vi "8-Axis (Producer Consumer - PC).vi"() -> ()   [LabVIEW 2013]
uses:
  Typedef/Typedef_Motor_Message.ctl
  EMC API/EMC_Typedef_Motor_Parameters.ctl
  Functional_Global/Typedef_Message_Queue_Action.ctl
  Globals/Global Stop.vi
  <vilib>/Motion/Express/_s/nimc.ex.clearFaults.clearFaults.axis.vi
  <vilib>/Motion/Express/_s/nimc.ex.power.power.axis.vi
  <vilib>/Motion/Express/_s/nimc.ex.resetPosition.resetPosition.axis.vi
  <vilib>/Motion/Express/_s/nimc.ex.read.readTrajectoryData.axis.vi
  <vilib>/Motion/BlockNode/FB.NIMotion.xnode
  Functional_Global/Typedef_FPGA_Interface_Action.ctl
panel:
  out "Command":T1={"Axis"="", "Motion Parameters"={"position"=1000.0, "velocity"=1000.0, "acceleration"=10000.0, "deceleration"=10000.0, "accel. jerk"=10000.0, "decel. jerk"=10000.0}}
  out "Message":string
  out "# elements in queue":i32
  out "error out":errorcluster
  out "Axis Positions":T3(graph)
  out "Axis Velocities":T3(graph)
  out "Array":dbl[](array[knob]) scale=0.0..1000.0
  in  "stop":bool
  # "This example demonstrates how to set up an multi-axis SW architecture using SoftMotion.  You can have state machines that \"produce\" the motion commands, and the consumer will then digest them one at a time.\n\nIn this example, 3 producer loops generate random motion commands at random times (within 1000ms each iteration.) This VI is also meant as a stress test to see if the SM engine is robust enough for complex sequences of motion commands."
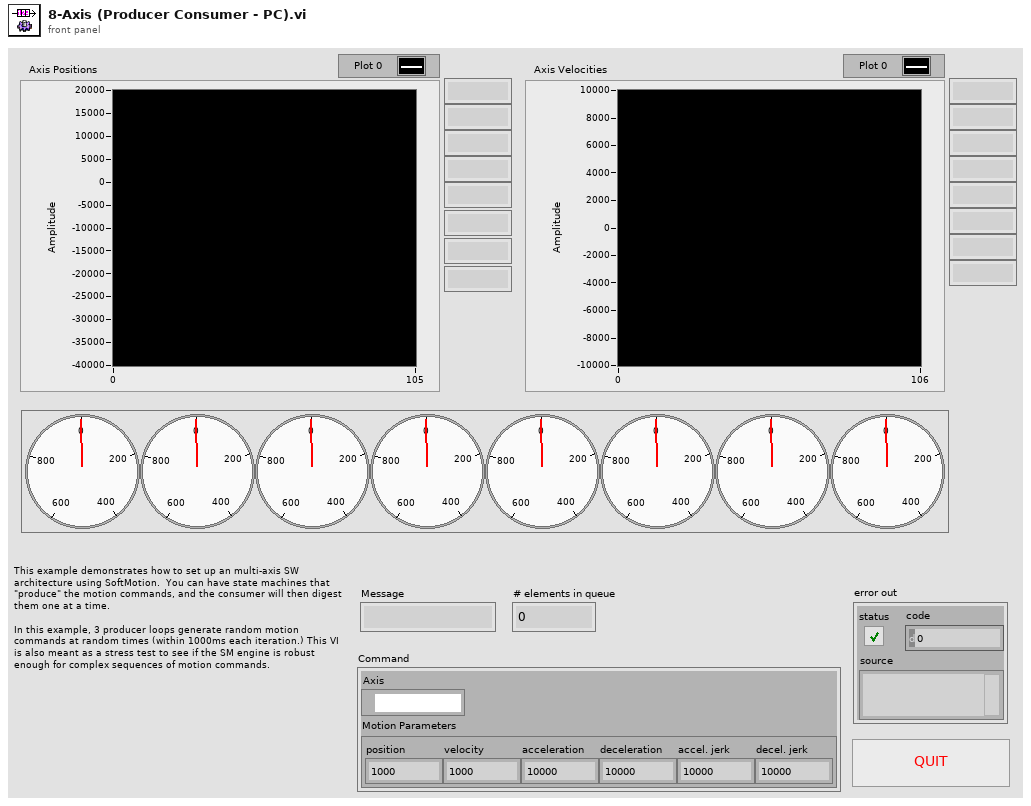
[diagram p1: front panel]
types:
  T1 = typedef "Typedef_Motor_Message.ctl" = cluster{"Axis":refnum<k21>, "Motion Parameters":T2}
  T2 = typedef "EMC_Typedef_Motor_Parameters.ctl" = cluster{"position":dbl, "velocity":dbl, "acceleration":dbl, "deceleration":dbl, "accel. jerk":dbl, "decel. jerk":dbl}
  T3 = cluster{"[0]":dbl, "[1]":dbl, "[2]":dbl, "[3]":dbl, "[4]":dbl, "[5]":dbl, "[6]":dbl, "[7]":dbl}
  T4 = typedef "Typedef_Message_Queue_Action.ctl" = enum16{"Init MQueue", "Get MQueue Ref", "Close MQueue"}
  T5 = typedef "Typedef_FPGA_Interface_Action.ctl" = enum16{"Initialize FPGA", "Get FPGA Reference", "Close FPGA"}
  T6 = typedef "Message Queue.lvlib/Message Cluster.ctl" = cluster{"Message":string, "Message Data":variant}
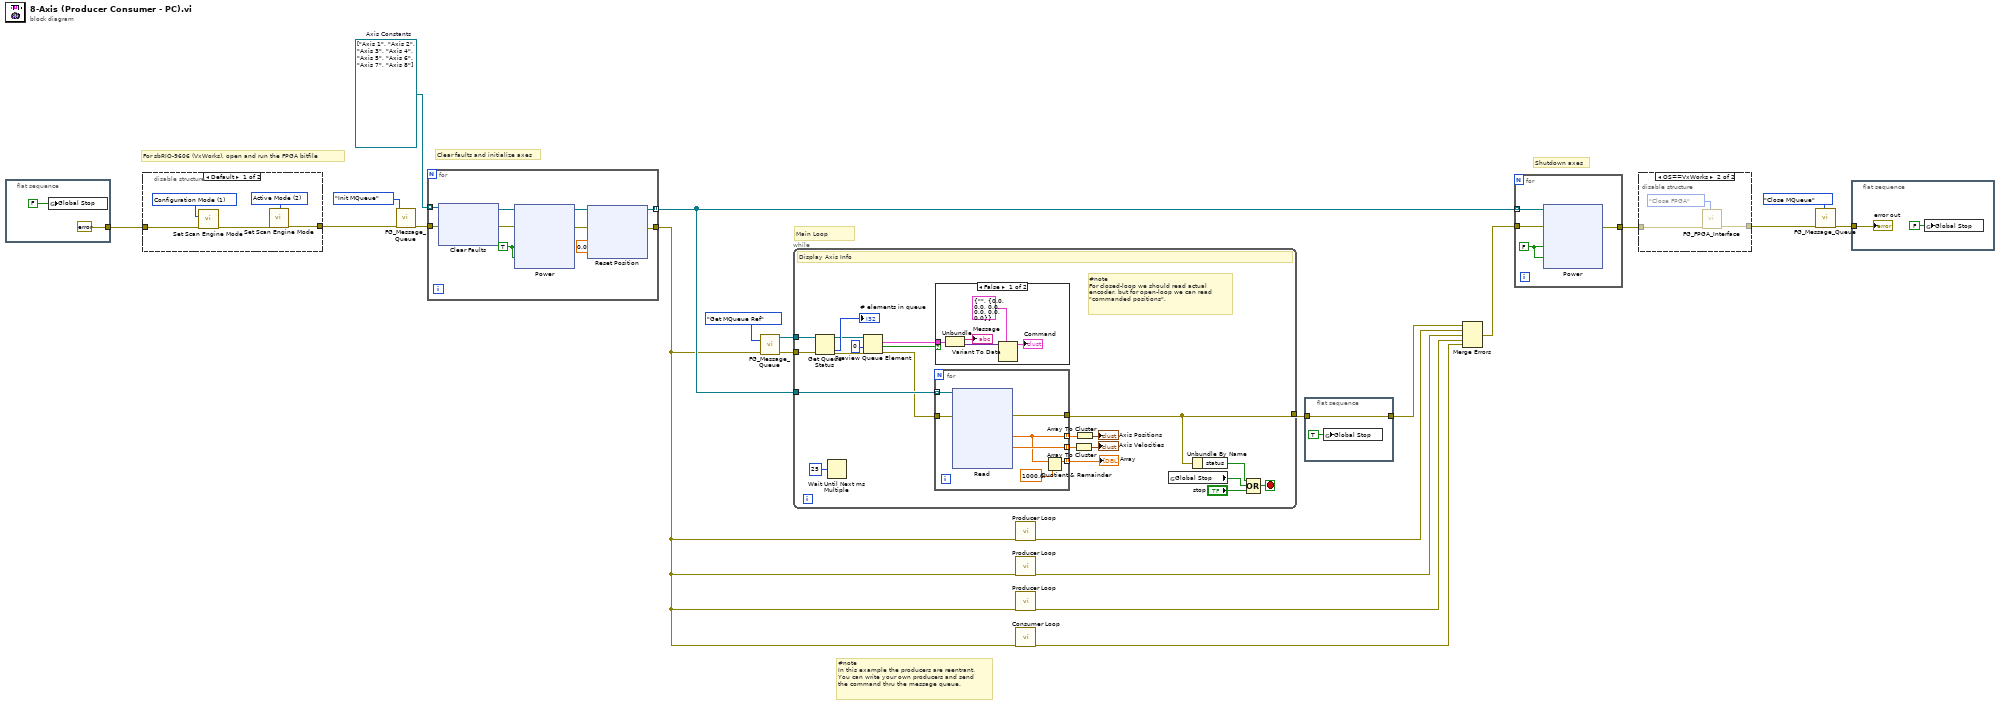
[diagram p0: block diagram]
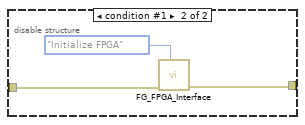
[diagram p3: hidden frame]
diagram:
  w20 = refnum<k21>[] ["Axis 1", "Axis 2", "Axis 3", "Axis 4", "Axis 5", "Axis 6", "Axis 7", "Axis 8"]  # Axis Constants
  # "#note\nIn this example the producers are reentrant.\nYou can write your own producers and send\nthe command thru the message queue."
  # "For sbRIO-9606 (VxWorks), open and run the FPGA bitfile"
  # "Shutdown axes"
  # "Main Loop"
  # "Clear faults and initialize axes"
  n1 = flat-sequence {
    tunnel: [errorcluster {"status"=FALSE, "code"=0, "source"=""} ("error in (no error)")] -> w21
    frame #0 {
      n2 = global write "Global Stop.vi" "Global Stop"(FALSE ("stop")) -> ()
    }
  }
  n3 = disable-structure shown="Default" {
    disable-tunnel: [w28 w29] -> w16
    disable-tunnel: w21 -> [w27 w30]
    frame condition #0 (active) {
      w24 = 1 items=["Configuration Mode"=1, "Active Mode"=2] ("mode (Active Mode)")
      w25 = 2 items=["Configuration Mode"=1, "Active Mode"=2] ("mode (Active Mode)")
      n4 = call <vilib>:"Set Scan Engine Mode.vi"("mode (Active Mode)"=w24, "error in (no error)"=w27) -> ("error out"=w26:errorcluster)  [unwired: 13 in]
      n5 = call <vilib>:"Set Scan Engine Mode.vi"("mode (Active Mode)"=w25, "error in (no error)"=w26) -> ("error out"=w28:errorcluster)  [unwired: 13 in]
    }
    frame condition #1 {
      n6 = call "FG_FPGA_Interface.vi"("Action"=Typedef_FPGA_Interface_Action."Initialize FPGA", "error in"=w30) -> ("error out"=w29:errorcluster)  [unwired: 8 in, 1 out]
    }
  }
  n7 = call "FG_Message_Queue.vi"("Action"=Typedef_Message_Queue_Action."Init MQueue", "error in"=w16) -> ("error out"=w15:errorcluster)  [unwired: 8 in, 1 out]
  n8 = for {
    tunnel: [w34] -> w2
    tunnel: [w32] -> w10 mode=indexing
    tunnel: w15 -> [w38]
    tunnel: w20 -> [w37] mode=indexing
    w41 = TRUE ("enable axis")
    n9 = xnode ("Clear Faults")("resource"=w37, "error in"=w38) -> ("resource out"=w39:refnum<k21>, "error out"=w40:errorcluster)
    n10 = xnode ("Power")("enable axis"=w41, "enable drive"=w41, "resource"=w39, "error in"=w40) -> ("resource out"=w33:refnum<k21>, "error out"=w35:errorcluster)
    n11 = xnode ("Reset Position")("position"=0.0, "resource"=w33, "error in"=w35) -> ("resource out"=w32:refnum<k21>, "error out"=w34:errorcluster)
  }
  n12 = call "FG_Message_Queue.vi"("Action"=Typedef_Message_Queue_Action."Get MQueue Ref", "error in"=w2) -> ("error out"=w1:errorcluster, "Message Queue"=w3:refnum<queue>)  [unwired: 8 in]
  n13 = while {
    tunnel: w1 -> [w68]
    tunnel: w10 -> [w78]
    tunnel: [w61] -> w18
    tunnel: w3 -> [w70]
    stop <- w71 stop-if-true
    # "#note \nFor closed-loop we should read actual \nencoder, but for open-loop we can read\n\"commanded positions\"."
    # "Display Axis Info"
    n14 = Get Queue Status(queue=w70, error in (no error)=w68) -> (queue out=w64:refnum<queue>, error out=w66:errorcluster, # elements in queue=→"# elements in queue":i32)  [unwired: 1 in, 5 out]
    n15 = Wait Until Next ms Multiple(millisecond multiple=u32 25) -> ()  [unwired: 1 out]
    n16 = Preview Queue Element(queue=w64, timeout in ms (-1)=0, error in (no error)=w66) -> (element=w63:T6, timed out?=w62:bool, error out=w65:errorcluster)  [unwired: 1 out]
    n17 = for {
      tunnel: [w93] -> w61
      tunnel: [w88] -> w76 mode=indexing
      tunnel: [w92] -> w81 mode=indexing
      tunnel: w65 -> [w91]
      tunnel: w78 -> [w90] mode=indexing
      tunnel: [w87] -> w77 mode=indexing
      n18 = xnode ("Read")("resource"=w90, "error in"=w91) -> ("commanded position"=w88:dbl, "commanded vel."=w92:dbl, "error out"=w93:errorcluster)  [unwired: 2 out]
      n19 = Quotient & Remainder(x=w88, y=1000.0) -> (x-y*floor(x/y)=w87:dbl)  [unwired: 1 out]
    }
    "Array" <- w77
    n20 = case shown="False" w62 {
      tunnel: w63 -> [w86 _]
      frame False {
        n21 = Unbundle(w86) -> ("Message"=→"Message":string, "Message Data"=w83:variant)
        n22 = Variant To Data(type=T1 {"Axis"="", "Motion Parameters"={"position"=0.0, "velocity"=0.0, "acceleration"=0.0, "deceleration"=0.0, "accel. jerk"=0.0, "decel. jerk"=0.0}} ("Motor_Message"), Variant=w83) -> (data=→"Command":T1)  [unwired: 1 in, 1 out]
      }
      frame True {
      }
    }
    n23 = Array To Cluster(array=w81) -> (cluster=→"Axis Velocities":T3)
    n24 = Array To Cluster(array=w76) -> (cluster=→"Axis Positions":T3)
    n25 = global read "Global Stop.vi" "Global Stop"() -> (w72:bool)
    n26 = Unbundle By Name(w61) -> ("status"=w73:bool)
    n27 = Compound Arithmetic op=OR(w73, w72, "stop") -> (w71:bool)
  }
  n28 = call "Producer Loop.vi"("error in (no error)"=w2) -> ("error out"=w6:errorcluster)  [unwired: 10 in]
  n29 = call "Producer Loop.vi"("error in (no error)"=w2) -> ("error out"=w5:errorcluster)  [unwired: 10 in]
  n30 = call "Producer Loop.vi"("error in (no error)"=w2) -> ("error out"=w8:errorcluster)  [unwired: 10 in]
  n31 = call "Consumer Loop.vi"("error in (no error)"=w2) -> ("error out"=w7:errorcluster)  [unwired: 10 in]
  n32 = flat-sequence {
    tunnel: w18 -> [w101]
    tunnel: [w101] -> w9
    frame #0 {
      n33 = global write "Global Stop.vi" "Global Stop"(TRUE ("stop")) -> ()
    }
  }
  n34 = Merge Errors(w9, w6, w5, w8, w7) -> (w14:errorcluster)
  n35 = for {
    tunnel: w10 -> [w106] mode=indexing
    tunnel: [w104] -> w19
    tunnel: w14 -> [w103]
    w105 = FALSE ("enable axis")
    n36 = xnode ("Power")("enable axis"=w105, "enable drive"=w105, "resource"=w106, "error in"=w103) -> ("error out"=w104:errorcluster)  [unwired: 1 out]
  }
  n37 = disable-structure shown="OS==VxWorks" {
    disable-tunnel: [w117 w118] -> w12
    disable-tunnel: w19 -> [w117 w119]
    frame condition #0 (active) {
    }
    frame condition #1 {
      n38 = call "FG_FPGA_Interface.vi"("Action"=Typedef_FPGA_Interface_Action."Close FPGA", "error in"=w119) -> ("error out"=w118:errorcluster)  [unwired: 8 in, 1 out]
    }
  }
  n39 = call "FG_Message_Queue.vi"("Action"=Typedef_Message_Queue_Action."Close MQueue", "error in"=w12) -> ("error out"=w11:errorcluster)  [unwired: 8 in, 1 out]
  n40 = flat-sequence {
    tunnel: w11 -> [w121]
    frame #0 {
      n41 = global write "Global Stop.vi" "Global Stop"(FALSE ("stop")) -> ()
      "error out" <- w121
    }
  }
